vi "WriteSLMPAttern.vi"(8 "Holo Array":T1[](array[typedef]) {"Modes"."Amplititute" step=0.05}, 11 "General settings":T2) -> (3 "Display Array":u8[][](array[numeric]))   [LabVIEW 2014]
uses:
  Controls/SLM General Settings.ctl
  Controls/Holo Controls.ctl
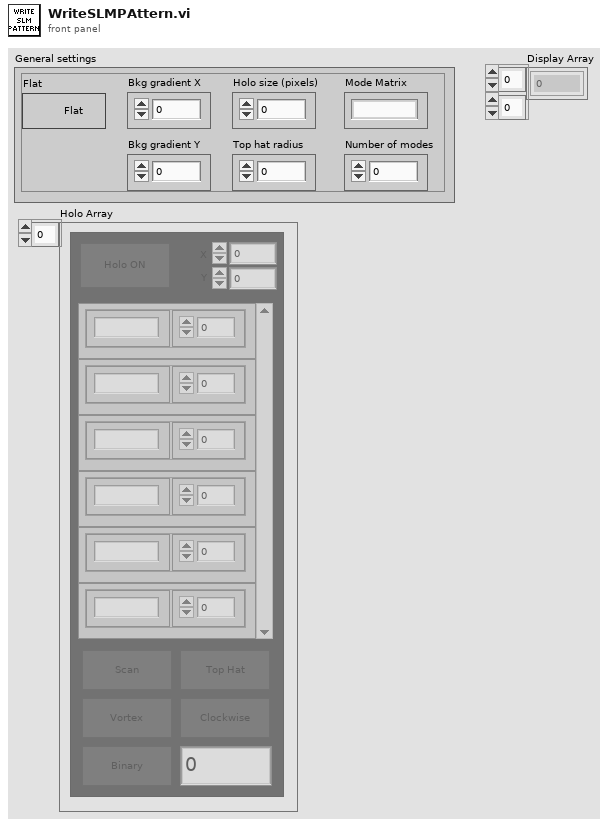
[diagram p1: front panel]
types:
  T1 = typedef "Holo Controls.ctl" = cluster{"Top Hat":bool, "Modes":cluster{"Mode ID":string, "Amplititute":dbl}[], "Vortex":bool, "Clockwise":bool, "X":dbl, "Y":dbl, "Holo ON":bool, "Scan":bool, "Binary":bool, "Binary Angle":dbl}
  T2 = typedef "SLM General Settings.ctl" = cluster{"Holo size (pixels)":i32, "Top hat radius":dbl, "Number of modes":i32, "Bkg gradient X":dbl, "Bkg gradient Y":dbl, "Flat":bool, "Mode Matrix":u16}
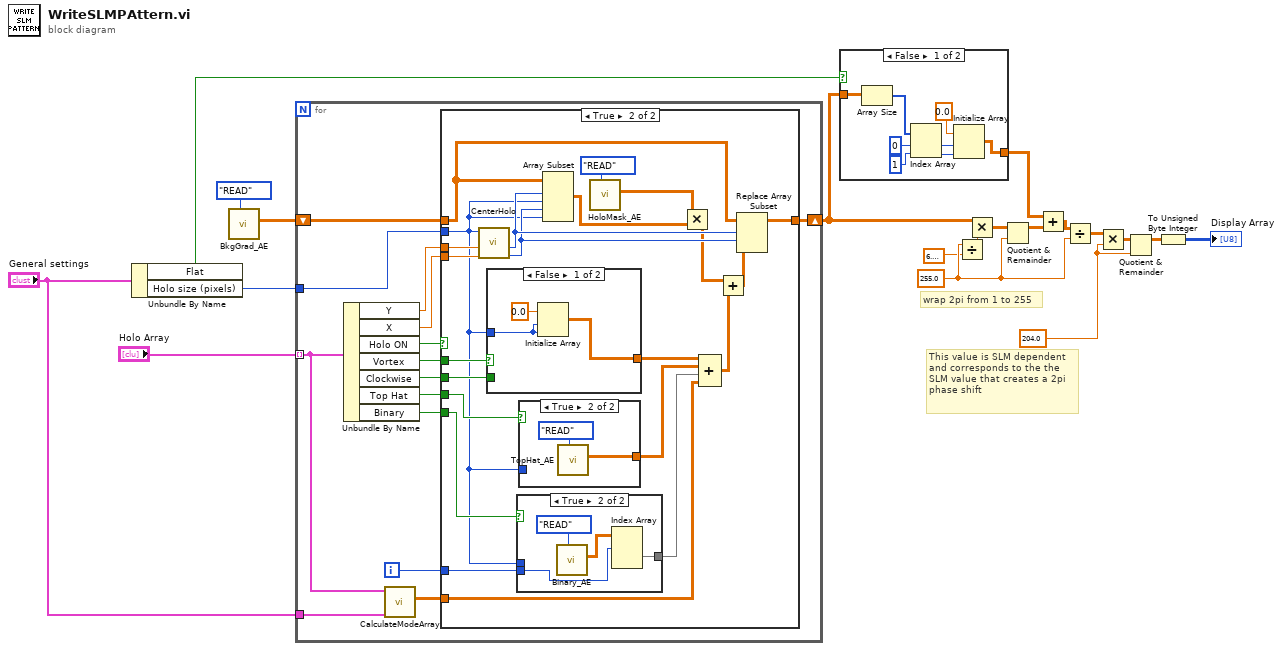
[diagram p0: block diagram]
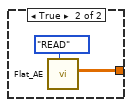
[diagram p2: hidden frame]
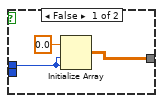
[diagram p4: hidden frame]
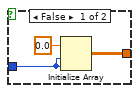
[diagram p5: hidden frame]
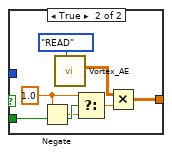
[diagram p6: hidden frame]
diagram:
  w19 = 204.0 ("Wrap Value")
  w13 = 255.0 ("y")
  # "This value is SLM dependent and corresponds to the the SLM value that creates a 2pi phase shift"
  # "wrap 2pi from 1 to 255"
  n1 = Unbundle By Name("General settings") -> ("Flat"=w9:bool, "Holo size (pixels)"=w1:i32)
  n2 = call "BkgGrad_AE.vi"("Action"=enum16{"READ", "WRITE"}."READ") -> ("BkgGrad Out"=w5:dbl[][])  [unwired: 10 in]
  n3 = for {
    tunnel: "Holo Array" -> [w23] mode=indexing
    tunnel: w1 -> [w29]
    shift-right: [w25] -> w2
    shift-left: w5 -> [w26]
    tunnel: "General settings" -> [w22]
    i -> [w20]
    n4 = Unbundle By Name(w23) -> ("Y"=w28:dbl, "X"=w27:dbl, "Holo ON"=w30:bool, "Vortex"=w33:bool, "Clockwise"=w32:bool, "Top Hat"=w31:bool, "Binary"=w21:bool)
    n5 = call "CalculateModeArray.vi"("General settings"=w22, "Holo Control"=w23) -> ("ModeArray"=w24:dbl[][])  [unwired: 9 in]
    n6 = case shown="True" w30 {
      tunnel: w33 -> [_ w52]
      tunnel: w32 -> [_ w56]
      tunnel: w26 -> [w34 w48]
      tunnel: w31 -> [_ w51]
      tunnel: w29 -> [_ w38]
      tunnel: w28 -> [_ w55]
      tunnel: w27 -> [_ w54]
      tunnel: [w34 w49] -> w25
      tunnel: w24 -> [_ w36]
      tunnel: w21 -> [_ w39]
      tunnel: w20 -> [_ w35]
      frame False {
      }
      frame True {
        n7 = call "CenterHolo.vi"("X"=w54, "Y"=w55, "Holo Size"=w38) -> ("X centered"=w46:i32, "Y centered"=w47:i32)  [unwired: 7 in]
        n8 = case shown="False" w52 {
          tunnel: w56 -> [_ w78]
          tunnel: [w70 w72] -> w45
          tunnel: w38 -> [w69 _]
          frame False {
            n9 = Initialize Array(0.0 ("element"), w69, w69) -> (w70:dbl[][])
          }
          frame True {
            w77 = 1.0 ("t")
            n10 = Negate(x=w77) -> (-x=w76:dbl)
            n11 = call "Vortex_AE.vi"("Action"=enum16{"READ", "WRITE"}."READ") -> ("Vortex Out"=w74:dbl[][])  [unwired: 10 in]
            n12 = Select(t=w77, s=w78, f=w76) -> (s? t:f=w73:dbl)
            n13 = Multiply(x=w74, y=w73) -> (x*y=w72:dbl[][])
          }
        }
        n14 = case shown="True" w39 {
          tunnel: [w58 w61] -> w37
          tunnel: w38 -> [w57 _]
          tunnel: w35 -> [_ w60]
          frame False {
            n15 = Initialize Array(0.0 ("element"), w57, w57) -> (w58:dbl[][])
          }
          frame True {
            n16 = call "Binary_AE.vi"("Action"=enum16{"READ", "WRITE"}."READ") -> ("BINARY Out"=w62:dbl[][][])  [unwired: 10 in]
            n17 = Index Array(array=w62, index (dim 0)=w60) -> (element=w61:dbl[][])  [unwired: 2 in]
          }
        }
        n18 = case shown="True" w51 {
          tunnel: [w65 w67] -> w50
          tunnel: w38 -> [w64 _]
          frame False {
            n19 = Initialize Array(0.0 ("element"), w64, w64) -> (w65:dbl[][])
          }
          frame True {
            n20 = call "TopHat_AE.vi"("Action"=enum16{"READ", "WRITE"}."READ") -> ("TopHat Out"=w67:dbl[][])  [unwired: 10 in]
          }
        }
        n21 = Array Subset(array=w48, index (row)=w47, length (row)=w38, index (col)=w46, length (col)=w38) -> (w40:dbl[][])
        n22 = call "HoloMask_AE.vi"("Action"=enum16{"READ", "WRITE"}."READ") -> ("HoloMask Out"=w41:dbl[][])  [unwired: 10 in]
        n23 = Multiply(x=w41, y=w40) -> (x*y=w44:dbl[][])
        n24 = Compound Arithmetic op=ADD(w45, w50, w37, w36) -> (w42:dbl[][])
        n25 = Add(x=w44, y=w42) -> (x+y=w43:dbl[][])
        n26 = Replace Array Subset(array=w48, new element=w43, index (row)=w47, index (col)=w46) -> (w49:dbl[][])
      }
    }
  }
  n27 = case shown="False" w9 {
    tunnel: [w79 w87] -> w11
    tunnel: w2 -> [w80 _]
    frame False {
      n28 = Array Size(array=w80) -> (size(s)=w82:i32[])
      n29 = Index Array(array=w82, index #1=0 ("index"), index #2=1 ("index")) -> (element #1=w84:i32, element #2=w85:i32)
      n30 = Initialize Array(0.0 ("element"), w84, w85) -> (w79:dbl[][])
    }
    frame True {
      n31 = call "Flat_AE.vi"("Action"=enum16{"READ", "WRITE"}."READ") -> ("Flat Out"=w87:dbl[][])  [unwired: 10 in]
    }
  }
  n32 = Divide(x=w13, y=6.283185307179586) -> (x/y=w7:dbl)
  n33 = Multiply(x=w2, y=w7) -> (x*y=w6:dbl[][])
  n34 = Quotient & Remainder(x=w6, y=w13) -> (x-y*floor(x/y)=w10:dbl[][])  [unwired: 1 out]
  n35 = Add(x=w11, y=w10) -> (x+y=w12:dbl[][])
  n36 = Divide(x=w12, y=w13) -> (x/y=w14:dbl[][])
  n37 = Multiply(x=w14, y=w19) -> (x*y=w15:dbl[][])
  n38 = Quotient & Remainder(x=w15, y=w19) -> (x-y*floor(x/y)=w16:dbl[][])  [unwired: 1 out]
  n39 = To Unsigned Byte Integer(number=w16) -> (unsigned 8bit integer=→"Display Array":u8[][])
